vi "SMU_Config_Pulsed_Current.vi"(0 "IVI Refnum in":refnum<k15>, 5 "error in (no error)":errorcluster, 8 "Current_Pulse_Parameters":T1={"Source Delay (Sec)"=0.0, "Pulse On Time (Sec)"=0.001, "Pulse Bias Delay (Sec)"=0.0, "Aperture Time (Sec)"=1.25e-05, "Pulse Off Time (Sec)"=5e-05, "Pulse Current Level Range"=0.0001, "Pulse Bias Current Level"=0.0, "Pulse Voltage Limit"=60.0, "Pulse Voltage Limit Range"=60.0, "Pulse Bias Voltage Limit"=60.0, "Pulse Current Level"=-2.4e-05} {"Pulse Current Level" format="%.5p"; "Pulse Bias Voltage Limit" format="%.5p"; "Pulse Voltage Limit Range" format="%#.6p"; "Pulse Voltage Limit" format="%.5p"; "Pulse Bias Current Level" format="%.5p"; "Pulse Current Level Range" format="%#.6p"; "Pulse Off Time (Sec)" format="%#_6p"; "Aperture Time (Sec)" format="%#_6p"; "Pulse Bias Delay (Sec)" format="%.3p"; "Pulse On Time (Sec)" format="%#_6p"; "Source Delay (Sec)" format="%.3p"}, 12 "Channel List":string) -> (14 "IVI Refnum out":refnum<k15>, 17 "Measurement:Measure Record Length":i32=39, 18 "Measurement:Aperture Time":dbl=1.2777777777777777e-05 format="%#_6p", 19 "error out":errorcluster)   [LabVIEW 2013]
uses:
  Controls/Current_Pulse_Parameters.ctl
  <instrlib>/niDCPower/nidcpower.llb/niDCPower Source Mode.ctl
  <instrlib>/niDCPower/nidcpower.llb/niDCPower Aperture Time Units.ctl
  <instrlib>/niDCPower/nidcpower.llb/niDCPower Output Function.ctl
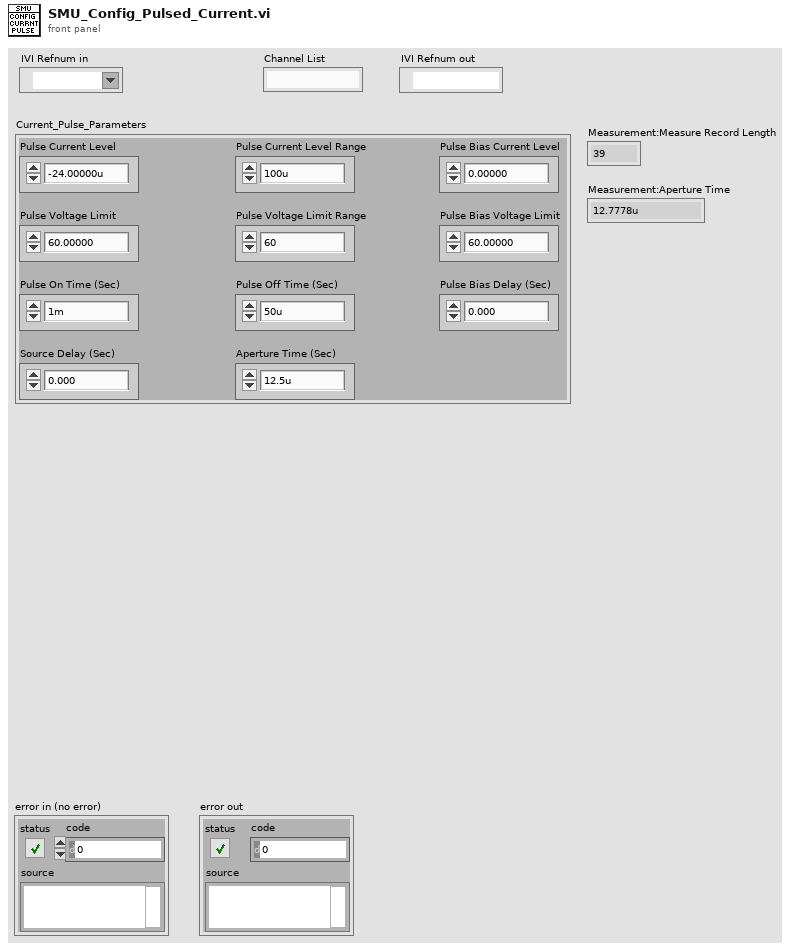
[diagram p1: front panel]
types:
  T1 = typedef "Current_Pulse_Parameters.ctl" = cluster{"Source Delay (Sec)":dbl, "Pulse On Time (Sec)":dbl, "Pulse Bias Delay (Sec)":dbl, "Aperture Time (Sec)":dbl, "Pulse Off Time (Sec)":dbl, "Pulse Current Level Range":dbl, "Pulse Bias Current Level":dbl, "Pulse Voltage Limit":dbl, "Pulse Voltage Limit Range":dbl, "Pulse Bias Voltage Limit":dbl, "Pulse Current Level":dbl}
  T2 = typedef "niDCPower Output Function.ctl" = i32
  T3 = typedef "niDCPower Aperture Time Units.ctl" = i32
  T4 = typedef "niDCPower Source Mode.ctl" = i32
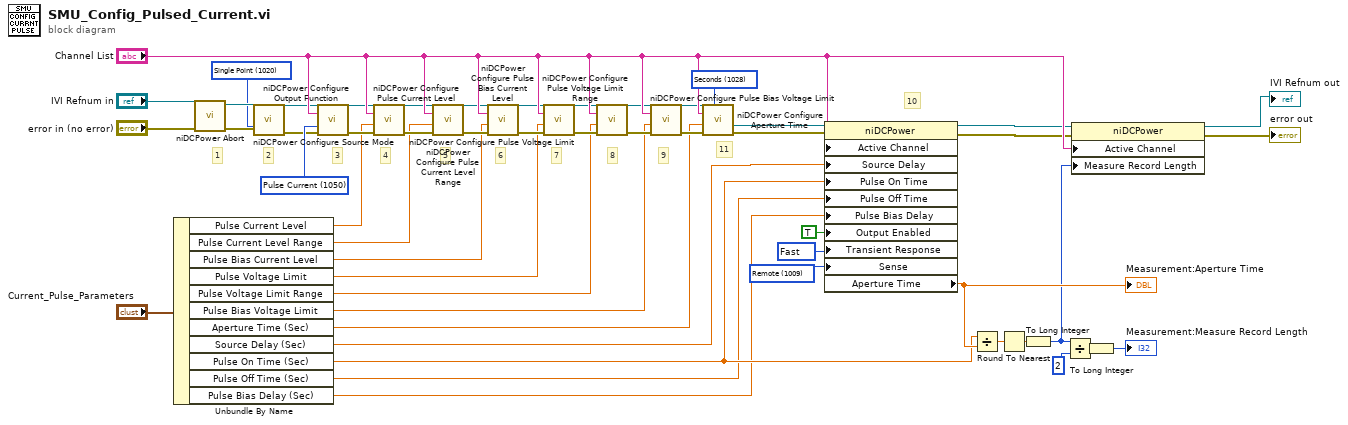
[diagram p0: block diagram]
diagram:
  w32 = 1009 items=["Local"=1008, "Remote"=1009] ("Measurement:Sense")
  w31 = 1039 items=["Slow"=1041, "Normal"=1038, "Fast"=1039, "Custom"=1042] ("Source:Transient Response")
  w26 = T2 1050 items=["DC Voltage"=1006, "DC Current"=1007, "Pulse Voltage"=1049, "Pulse Current"=1050] ("output function")
  w16 = T3 1028 items=["Seconds"=1028, "Powerline Cycles"=1029] ("aperture time units")
  w13 = T4 1020 items=["Single Point"=1020, "Sequence"=1021] ("source mode")
  # "9"
  # "8"
  # "7"
  # "6"
  # "5"
  # "4"
  # "3"
  # "11"
  # "10"
  # "2"
  # "1"
  n1 = Unbundle By Name("Current_Pulse_Parameters") -> ("Pulse Current Level"=w11:dbl, "Pulse Current Level Range"=w10:dbl, "Pulse Bias Current Level"=w9:dbl, "Pulse Voltage Limit"=w8:dbl, "Pulse Voltage Limit Range"=w7:dbl, "Pulse Bias Voltage Limit"=w6:dbl, "Aperture Time (Sec)"=w5:dbl, "Source Delay (Sec)"=w4:dbl, "Pulse On Time (Sec)"=w3:dbl, "Pulse Off Time (Sec)"=w2:dbl, "Pulse Bias Delay (Sec)"=w1:dbl)
  n2 = call <instrlib>:"niDCPower Abort.vi"("error in (no error)"="error in (no error)", "instrument handle"="IVI Refnum in") -> ("error out"=w44:errorcluster, "instrument handle out"=w45:refnum<k15>)  [unwired: 8 in]
  n3 = call <instrlib>:"niDCPower Configure Source Mode.vi"("error in (no error)"=w44, "source mode"=w13, "instrument handle"=w45) -> ("error out"=w15:errorcluster, "instrument handle out"=w14:refnum<k15>)  [unwired: 7 out]
  n4 = call <instrlib>:"niDCPower Configure Output Function.vi"("error in (no error)"=w15, "output function"=w26, "channel name"="Channel List", "instrument handle"=w14) -> ("error out"=w27:errorcluster, "instrument handle out"=w28:refnum<k15>)  [unwired: 6 out]
  n5 = call <instrlib>:"niDCPower Configure Pulse Current Level.vi"("error in (no error)"=w27, "pulse current level"=w11, "channel name"="Channel List", "instrument handle"=w28) -> ("error out"=w17:errorcluster, "instrument handle out"=w29:refnum<k15>)  [unwired: 6 in]
  n6 = call <instrlib>:"niDCPower Configure Pulse Current Level Range.vi"("error in (no error)"=w17, "pulse current level range"=w10, "channel name"="Channel List", "instrument handle"=w29) -> ("error out"=w18:errorcluster, "instrument handle out"=w19:refnum<k15>)  [unwired: 6 in]
  n7 = call <instrlib>:"niDCPower Configure Pulse Bias Current Level.vi"("error in (no error)"=w18, "pulse bias current level"=w9, "channel name"="Channel List", "instrument handle"=w19) -> ("error out"=w20:errorcluster, "instrument handle out"=w21:refnum<k15>)  [unwired: 6 in]
  n8 = call <instrlib>:"niDCPower Configure Pulse Voltage Limit.vi"("error in (no error)"=w20, "pulse voltage limit"=w8, "channel name"="Channel List", "instrument handle"=w21) -> ("error out"=w22:errorcluster, "instrument handle out"=w23:refnum<k15>)  [unwired: 6 in]
  n9 = call <instrlib>:"niDCPower Configure Pulse Voltage Limit Range.vi"("error in (no error)"=w22, "pulse voltage limit range"=w7, "channel name"="Channel List", "instrument handle"=w23) -> ("error out"=w24:errorcluster, "instrument handle out"=w25:refnum<k15>)  [unwired: 6 in]
  n10 = call <instrlib>:"niDCPower Configure Pulse Bias Voltage Limit.vi"("error in (no error)"=w24, "pulse bias voltage limit"=w6, "channel name"="Channel List", "instrument handle"=w25) -> ("error out"=w33:errorcluster, "instrument handle out"=w34:refnum<k15>)  [unwired: 6 in]
  n11 = call <instrlib>:"niDCPower Configure Aperture Time.vi"("aperture time units"=w16, "error in (no error)"=w33, "aperture time"=w5, "channel name"="Channel List", "instrument handle"=w34) -> ("error out"=w35:errorcluster, "instrument handle out"=w36:refnum<k15>)  [unwired: 5 in]
  n12 = property class="niDCPower"(reference=w36, error in=w35, "Active Channel"="Channel List", "Source Delay"=w4, "Pulse On Time"=w3, "Pulse Off Time"=w2, "Pulse Bias Delay"=w1, "Output Enabled"=TRUE ("Source:Output Enabled"), "Transient Response"=w31, "Sense"=w32) -> (reference out=w40:refnum<k15>, error out=w39:errorcluster, "Aperture Time"=w49:dbl)
  "Measurement:Aperture Time" <- w49
  n13 = Divide(x=w3, y=w49) -> (x/y=w41:dbl)
  n14 = Round To Nearest(number=w41) -> (nearest integer value=w42:dbl)
  n15 = To Long Integer(number=w42) -> (32bit integer=w46:i32)
  n16 = Divide(x=w46, y=2) -> (x/y=w47:dbl)
  n17 = property class="niDCPower"(reference=w40, error in=w39, "Active Channel"="Channel List", "Measure Record Length"=w46) -> (reference out=→"IVI Refnum out":refnum<k15>, error out=→"error out":errorcluster)
  n18 = To Long Integer(number=w47) -> (32bit integer=→"Measurement:Measure Record Length":i32)
